vi "GetParam.vi"(8 "error in (no error)":errorcluster caption="entrée d'erreur (pas d'erreur)", 11 "LeavePGroupsOut.lvclass":refnum<class "LeavePGroupsOut.lvclass">) -> (0 "error out":errorcluster caption="sortie d'erreur", 2 "LeavePGroupsOut":cluster{"n_groups":i32}={"n_groups"=2}, 3 "LeavePGroupsOut.lvclass":refnum<class "LeavePGroupsOut.lvclass">)   [LabVIEW 2020, in "LeavePGroupsOut.lvclass"]
doc: "Get Parameters"
uses:
  LeavePGroupsOut.lvclass
  LeavePGroupsOut.lvclass/LeavePGroupsOut.ctl
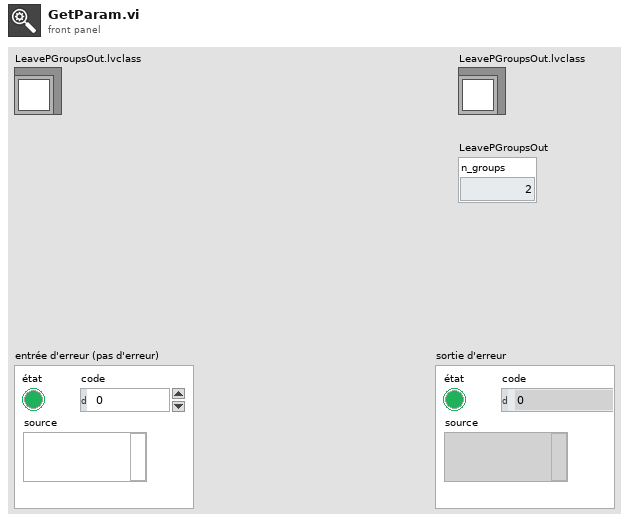
[diagram p1: front panel]
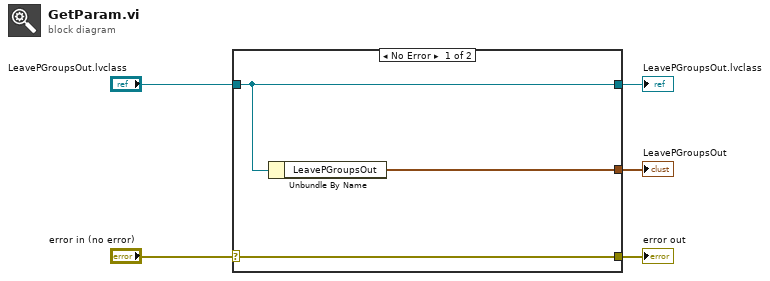
[diagram p0: block diagram]
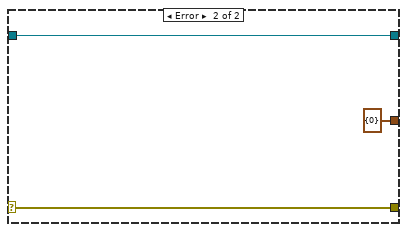
[diagram p2: hidden frame]
diagram:
  n1 = case shown="No Error" "error in (no error)" {
    selector: "error in (no error)" -> [w8 w10]
    tunnel: [w8 w10] -> w4
    tunnel: [w7 w11] -> w2
    tunnel: "LeavePGroupsOut.lvclass" -> [w7 w11]
    tunnel: [w6 cluster{"n_groups":i32} {"n_groups"=0} ("LeavePGroupsOut")] -> w1
    frame No Error {
      n2 = Unbundle By Name(w7) -> ("LeavePGroupsOut"=w6:cluster{"n_groups":i32})
    }
    frame Error {
    }
  }
  "error out" <- w4
  "LeavePGroupsOut.lvclass" <- w2
  "LeavePGroupsOut" <- w1
